vi "svx_Colormap Property Dialog.vi"(5 "Color Map in":refnum<vi>, 6 "Action In":T4, 7 "Refnum":refnum<vi>, 8 "Cursor Lines only?":bool, 9 "Found Speed":bool, 10 "Data In":T2 {"Y scale"."multiplier" format="%.2f"; "Y scale"."offset" format="%.2f"; "X scale"."multiplier" format="%.2f"; "X scale"."offset" format="%.2f"; "spectral map" format="%.2f"}, 11 "State in":T1={"RefQueue"=refnum, "Properties/Undo"=refnum, "Bound"={"Width"=0, "Height"=0}, "Plot Area:Colors"={"FG Color"=11776947, "BG Color"=0}, "scale legend visible?"=FALSE, "graph palette visible?"=FALSE, "cursor palette visible?"=FALSE, "Ignore Array"=TRUE, "Smooth Update"=FALSE, "Z Scale"={"Z Scale.Scale Fit"=2, "Z Scale.Name Label.Text"="Amplitude", "Z Scale.Interpolate Color"=TRUE, "Visible"=TRUE, "Label Visible"=TRUE, "format string"="%#.2g", "Z Scale.Range"={"Minimum"=0.0, "Maximum"=500.0}}, "X Scale"={"X Scale.Scale Fit"=2, "X Scale.Offset and Multiplier"={"Offset"=0.0, "Multiplier"=1.0}, "X Scale.Name Label.Text"="Time", "X Scale.Range"={"Minimum"=0.0, "Maximum"=10.0}, "Visible"=TRUE, "Label Visible"=TRUE, "format string"="%#.2g"}, "Y Scale"={"Y Scale.Scale Fit"=2, "Y Scale.Offset and Multiplier"={"Offset"=0.0, "Multiplier"=1.0}, "Y Scale.Name Label.Text"="Frequency", "Y Scale.Range"={"Minimum"=0.0, "Maximum"=500.0}, "Visible"=TRUE, "Label Visible"=TRUE, "format string"="%#.2g"}, "Annotation List"=[], "Cursor List"=[], "Display Frequency Lines"=TRUE, "Display Order Lines"=TRUE, "Display Order text"=TRUE, "Display Frequency text"=TRUE, "Order Lineproperty"={"Line"={"Width"=1, "Style"=enum."Dash"}, "color"=0}, "Order Textproperty"={"Test size"=11, "color"=16777222, "background"=16777216}, "Orders"=[], "Frequency"=[], "Frequency Lineproperty"={"Line"={"Width"=1, "Style"=enum."Dash"}, "color"=0}, "Frequency Textproperty"={"Test size"=11, "color"=16777222, "background"=16777216}, "Display Order from Cursor"=FALSE, "Display Freq from Cursor"=FALSE, "Active Cursor"=0, "Selected Cursors"=[], "Cursor Move"=refnum, "Scale Range Change"=refnum}) -> (3 "State out":T1={"RefQueue"=refnum, "Properties/Undo"=refnum, "Bound"={"Width"=0, "Height"=0}, "Plot Area:Colors"={"FG Color"=11776947, "BG Color"=0}, "scale legend visible?"=FALSE, "graph palette visible?"=FALSE, "cursor palette visible?"=FALSE, "Ignore Array"=TRUE, "Smooth Update"=FALSE, "Z Scale"={"Z Scale.Scale Fit"=2, "Z Scale.Name Label.Text"="Amplitude", "Z Scale.Interpolate Color"=TRUE, "Visible"=TRUE, "Label Visible"=TRUE, "format string"="%#.2g", "Z Scale.Range"={"Minimum"=0.0, "Maximum"=500.0}}, "X Scale"={"X Scale.Scale Fit"=2, "X Scale.Offset and Multiplier"={"Offset"=0.0, "Multiplier"=1.0}, "X Scale.Name Label.Text"="Time", "X Scale.Range"={"Minimum"=0.0, "Maximum"=10.0}, "Visible"=TRUE, "Label Visible"=TRUE, "format string"="%#.2g"}, "Y Scale"={"Y Scale.Scale Fit"=2, "Y Scale.Offset and Multiplier"={"Offset"=0.0, "Multiplier"=1.0}, "Y Scale.Name Label.Text"="Frequency", "Y Scale.Range"={"Minimum"=0.0, "Maximum"=500.0}, "Visible"=TRUE, "Label Visible"=TRUE, "format string"="%#.2g"}, "Annotation List"=[], "Cursor List"=[], "Display Frequency Lines"=TRUE, "Display Order Lines"=TRUE, "Display Order text"=TRUE, "Display Frequency text"=TRUE, "Order Lineproperty"={"Line"={"Width"=1, "Style"=enum."Dash"}, "color"=0}, "Order Textproperty"={"Test size"=11, "color"=16777222, "background"=16777216}, "Orders"=[], "Frequency"=[], "Frequency Lineproperty"={"Line"={"Width"=1, "Style"=enum."Dash"}, "color"=0}, "Frequency Textproperty"={"Test size"=11, "color"=16777222, "background"=16777216}, "Display Order from Cursor"=FALSE, "Display Freq from Cursor"=FALSE, "Active Cursor"=0, "Selected Cursors"=[], "Cursor Move"=refnum, "Scale Range Change"=refnum}, 4 "Action":T4)   [LabVIEW 2017, in "SVX Colormap.xctl"]
uses:
  <vilib>/addons/_XControls/Colormap/SVX Colormap.xctl
  <vilib>/_xctls/Action.ctl
  <vilib>/addons/_XControls/Colormap/subVIs/svx_Colormap Data.ctl
  <vilib>/addons/_XControls/Colormap/subVIs/svx_Colormap State.ctl
  <vilib>/addons/_XControls/Colormap/TypeDef/svx_Colormap_InnerState.ctl
  <vilib>/addons/_XControls/Colormap/TypeDef/svx_Colormap_Event.ctl
  <vilib>/_xctls/XControlSupport.lvlib
panel:
  in  "Autoscale flag":bool
  in  "Menu":T3(array[cluster])=[{"menu tag"="", "item names"="Delete Element", "item tags"="USER_SC_DELETE_ELEMENT"}, {"menu tag"="", "item names"="Delete All", "item tags"="USER_SC_DELETE_ALL"}]
  in  "Main Tab":T5(tab)
  in  "Enable State":T6(radio)
  in  "Caption":string="Colormap"
  in  "Label Text":string="Colormap"
  in  "Caption":bool
  in  "Label":bool=TRUE
  in  "Apply to":u16(ring) items=["X-Axis", "Y-Axis", "Z-Axis"]
  in  "Hide trailing zeros":bool
  in  "Digits":u8=1
  in  "Precision Type":u16(ring) items=["Digits of precision", "Significant digits"]
  in  "Type":i32(listbox)
  in  "Show scale":bool
  in  "Show scale label":bool
  in  "Axes":u16(ring) items=["X-Axis", "Y-Axis", "Z-Axis"]
  in  "Interpolate color":bool
  in  "Maximum":dbl
  in  "Minimum":dbl
  in  "Autoscale":bool
  in  "Name":string="Time"
  in  "Frequencies":dbl[](array[numeric])
  in  "Orders":dbl[](array[numeric])
  in  "Line Type":u16(ring) items=["Order Lines", "Frequency Lines"]
  in  "DisplayLines":bool
  in  "Displaytext":bool
  in  "Style":T7(ring)=enum."Dash"
  in  "Line width":u16=1 min=1
  in  "Line color":u32(colorbox)
  in  "Size":i16=10 min=1
  in  "Text color":u32(colorbox)=16777222
  in  "BG color":u32(colorbox)=16777216
  in  "Tip strip":string
  in  "Description":string
  in  "Help":bool
  in  "Cancel":bool
  in  "OK":bool
  # "Label"
  # "Caption"
  # "Enabled State"
  # "Line Settings"
  # "Text Settings"
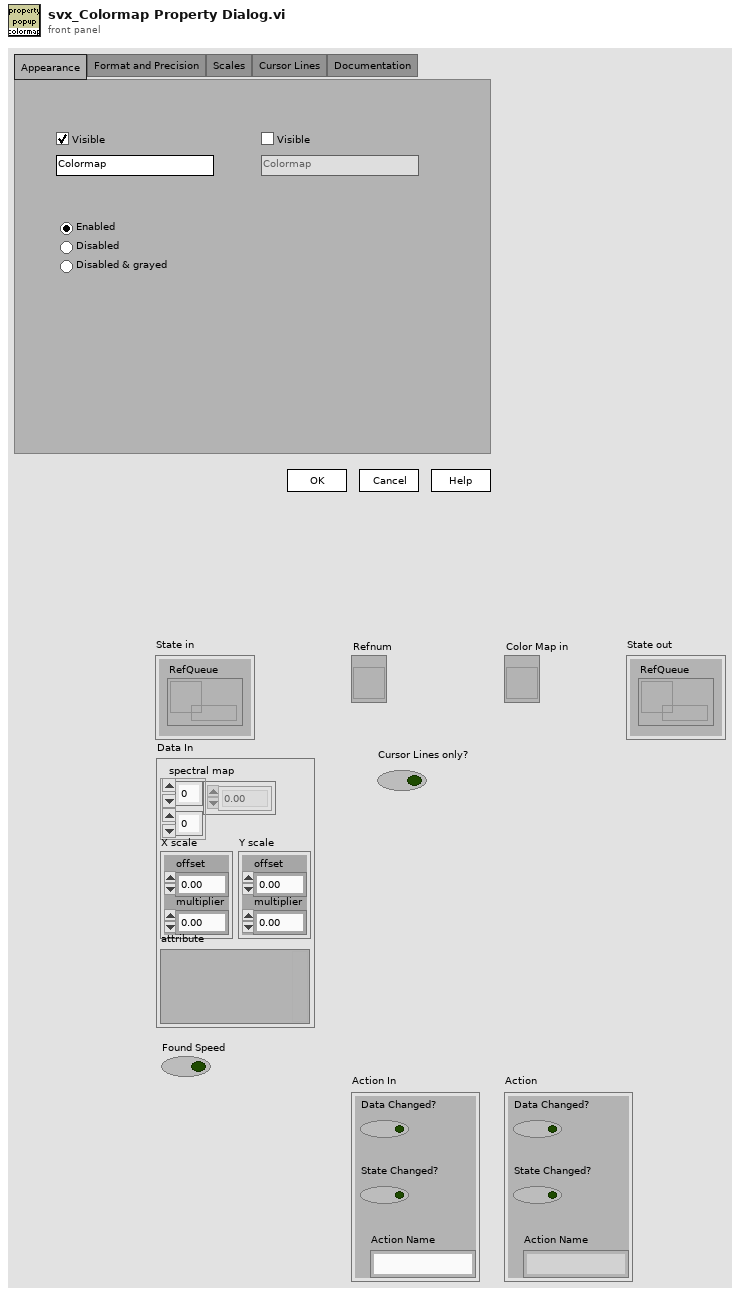
[diagram p1: front panel]
types:
  T1 = typedef "SVX Colormap.xctl/svx_Colormap State.ctl" = cluster{"RefQueue":refnum<queue>, "Properties/Undo":refnum<queue>, "Bound":cluster{"Width":u32, "Height":u32}, "Plot Area:Colors":cluster{"FG Color":u32, "BG Color":u32}, "scale legend visible?":bool, "graph palette visible?":bool, "cursor palette visible?":bool, "Ignore Array":bool, "Smooth Update":bool, "Z Scale":cluster{"Z Scale.Scale Fit":u8, "Z Scale.Name Label.Text":string, "Z Scale.Interpolate Color":bool, "Visible":bool, "Label Visible":bool, "format string":string, "Z Scale.Range":cluster{"Minimum":dbl, "Maximum":dbl}}, "X Scale":cluster{"X Scale.Scale Fit":u8, "X Scale.Offset and Multiplier":cluster{"Offset":dbl, "Multiplier":dbl}, "X Scale.Name Label.Text":string, "X Scale.Range":cluster{"Minimum":dbl, "Maximum":dbl}, "Visible":bool, "Label Visible":bool, "format string":string}, "Y Scale":cluster{"Y Scale.Scale Fit":u8, "Y Scale.Offset and Multiplier":cluster{"Offset":dbl, "Multiplier":dbl}, "Y Scale.Name Label.Text":string, "Y Scale.Range":cluster{"Minimum":dbl, "Maximum":dbl}, "Visible":bool, "Label Visible":bool, "format string":string}, "Annotation List":cluster{"Name":string, "Color":u32, "Style":u8, "Point Style":u8, "Name Visible":bool, "Allow Drag":bool, "Annotation Mode":u32, "Plot":i32, "Index":i32, "Position":cluster{"X":dbl, "Y":dbl}, "X Scale":u32, "Y Scale":u32, "Show Arrow":bool, "Lock Name":bool, "Plot Area":i32, "Label Offset":cluster{"X":dbl, "Y":dbl}}[], "Cursor List":cluster{"Name":string, "Color":u32, "Style":u8, "Point Style":u8, "Name Visible":bool, "Allow Drag":bool, "Cursor Mode":u32, "Plot":i32, "Index":i32, "Position":cluster{"X":dbl, "Y":dbl}, "X Scale":u32, "Y Scale":u32, "Watch Plots":i32[], "Watch All Plots":bool, "Plot Area":i32, "Label Offset":cluster{"X":dbl, "Y":dbl}}[], "Display Frequency Lines":bool, "Display Order Lines":bool, "Display Order text":bool, "Display Frequency text":bool, "Order Lineproperty":cluster{"Line":cluster{"Width":u16, "Style":enum32{"Solid", "Dash", "Dot", "DashDot", "DashDotDot"}}, "color":u32}, "Order Textproperty":cluster{"Test size":i16, "color":u32, "background":u32}, "Orders":dbl[], "Frequency":dbl[], "Frequency Lineproperty":cluster{"Line":cluster{"Width":u16, "Style":enum32{"Solid", "Dash", "Dot", "DashDot", "DashDotDot"}}, "color":u32}, "Frequency Textproperty":cluster{"Test size":i16, "color":u32, "background":u32}, "Display Order from Cursor":bool, "Display Freq from Cursor":bool, "Active Cursor":u32, "Selected Cursors":u32[], "Cursor Move":refnum<user-event>, "Scale Range Change":refnum<user-event>}
  T2 = typedef "SVX Colormap.xctl/svx_Colormap Data.ctl" = cluster{"spectral map":dbl[][], "X scale":cluster{"offset":dbl, "multiplier":dbl}, "Y scale":cluster{"offset":dbl, "multiplier":dbl}, "attribute":variant}
  T3 = cluster{"menu tag":string, "item names":string, "item tags":string}[]
  T4 = typedef "XControlSupport.lvlib/Action.ctl" = cluster{"Data Changed?":bool, "State Changed?":bool, "Action Name":string}
  T5 = enum32{"Appearance", "Format and Precision", "Scales", "Cursor Lines", "Documentation"}
  T6 = enum32{"Enabled", "Disabled", "Disabled & grayed"}
  T7 = enum32{"Solid", "Dash", "Dot", "DashDot", "DashDotDot"}
  T8 = cluster{"Label.Text":string, "Caption.Text":string, "Label.Visible":bool, "Caption.Visible":bool, "Disabled":u8, "Desc":string, "TipStrip":string}
  T9 = cluster{"Test size":i16, "color":u32, "background":u32}
  T10 = cluster{"Line":cluster{"Width":u16, "Style":enum32{"Solid", "Dash", "Dot", "DashDot", "DashDotDot"}}, "color":u32}
  T11 = typedef "SVX Colormap.xctl/svx_Colormap_Event.ctl" = enum16{"None", "[Axis] X Range", "[Axis] Y Range", "[Axis] Z Range", "[Axis] Range", "[Axis] X FString", "[Axis] Y FString", "[Axis] Z FString", "[Axis] X Name", "[Axis] X ScaleVis", "[Axis] X NameVis", "[Axis] Y Name", "[Axis] Y ScaleVis", "[Axis] Y NameVis", "[Axis] Z Name", "[Axis] Z ScaleVis", "[Axis] Z NameVis", "[Image] Line", "[Axis] Z Interp", "[Data] Update", "[Layout] Resize", "[ColorTable] Ignore Array", "[Legend] ScaleVis", "[Legend] GPVis", "[Legend] CPVis", "[Smooth] Update", "[Cursor] Update", "[Plot Area] Colors", "[Size] Minimum", "[Annotation] Update", "[Properties Dialog]", "[Axis] Autoscale X", "[Axis] Autoscale Y", "[Axis] Autoscale Z"}
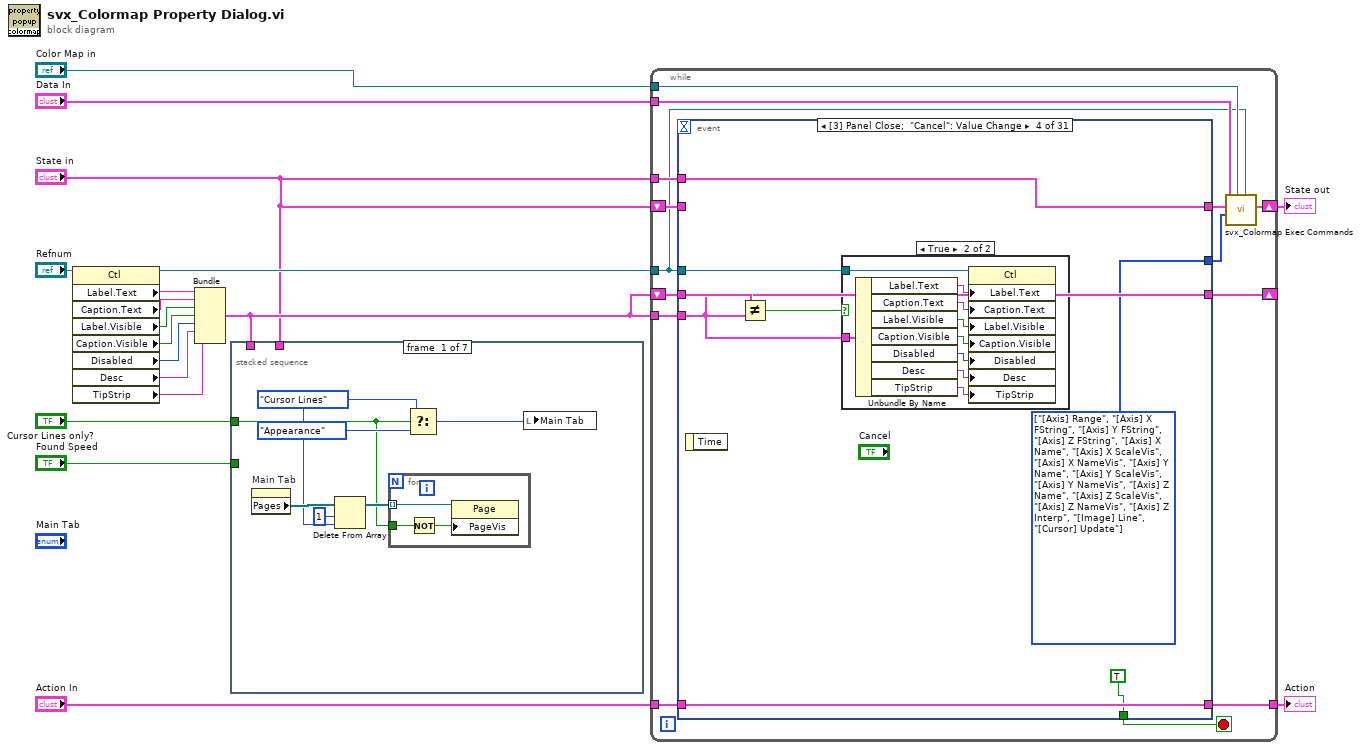
[diagram p0: block diagram]
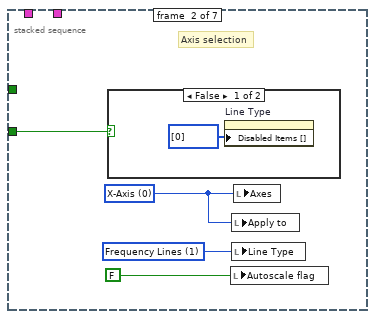
[diagram p2: hidden frame]
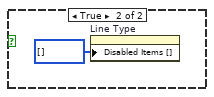
[diagram p3: hidden frame]
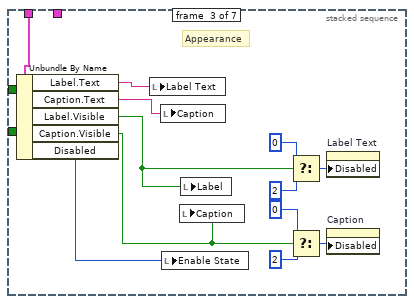
[diagram p4: hidden frame]
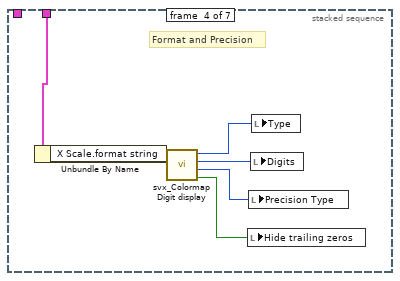
[diagram p5: hidden frame]
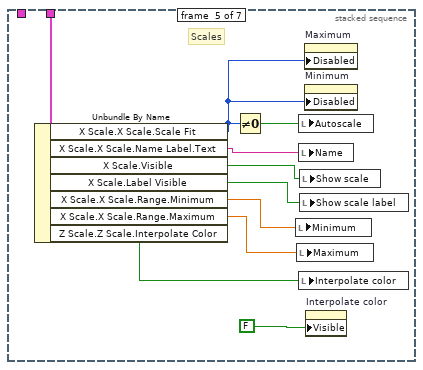
[diagram p6: hidden frame]
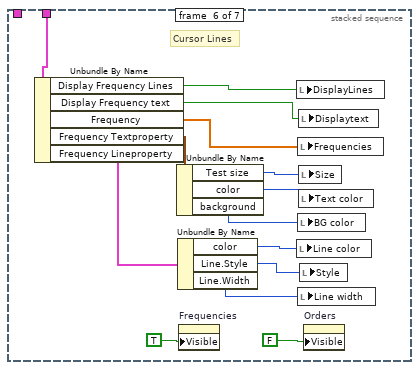
[diagram p7: hidden frame]
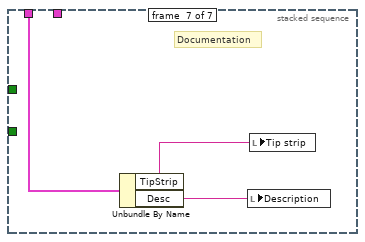
[diagram p8: hidden frame]
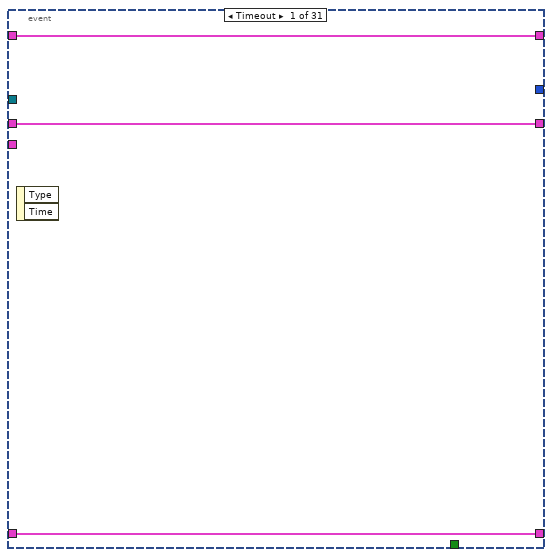
[diagram p9: hidden frame]
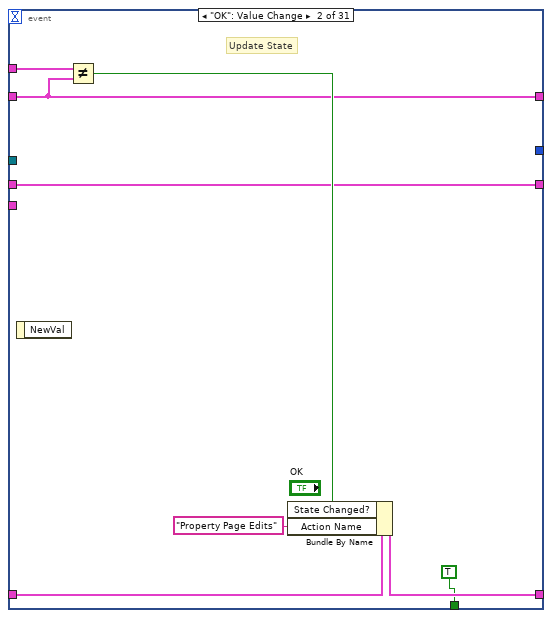
[diagram p10: hidden frame]
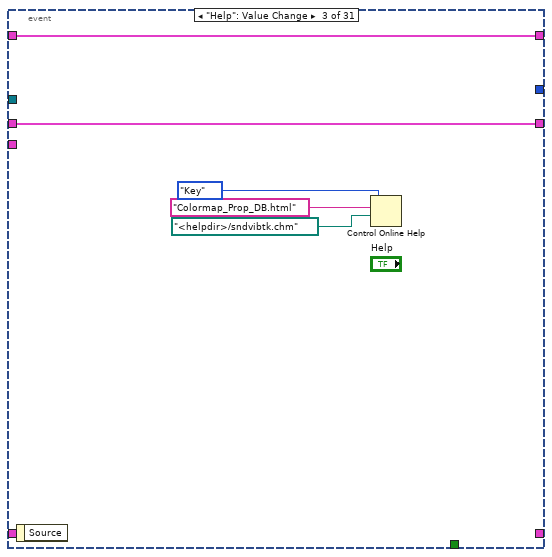
[diagram p11: hidden frame]
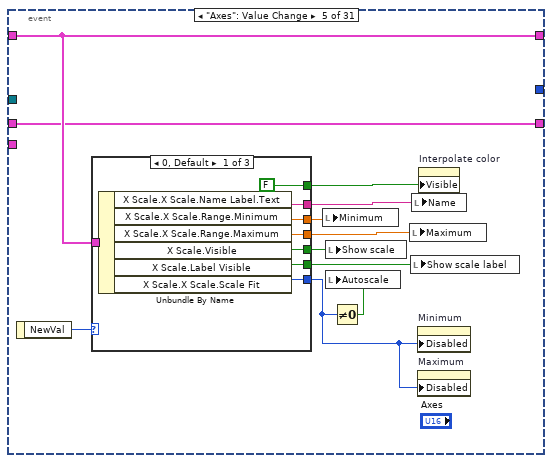
[diagram p13: hidden frame]
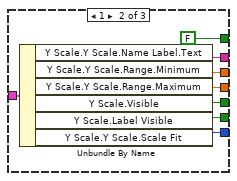
[diagram p14: hidden frame]
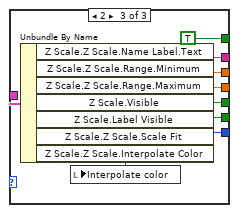
[diagram p15: hidden frame]
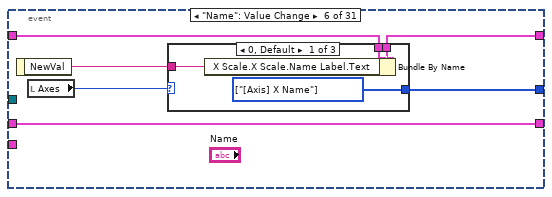
[diagram p16: hidden frame]
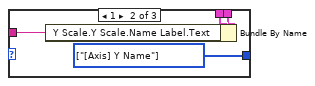
[diagram p17: hidden frame]
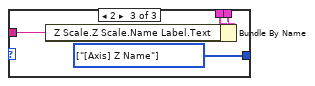
[diagram p18: hidden frame]
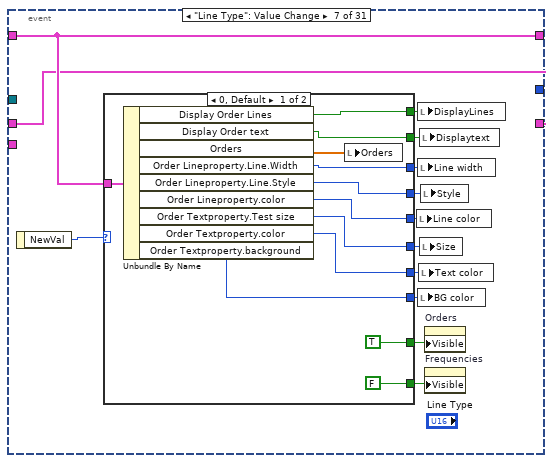
[diagram p19: hidden frame]
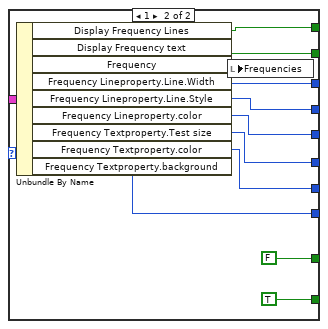
[diagram p20: hidden frame]
diagram:
  n1 = property class="Ctl"(reference="Refnum") -> (reference out=w14:refnum<vi>, "Label.Text"=w13:string, "Caption.Text"=w12:string, "Label.Visible"=w11:bool, "Caption.Visible"=w10:bool, "Disabled"=w9:u8, "Desc"=w8:string, "TipStrip"=w7:string)  [unwired: 1 in, 1 out]
  n2 = Bundle("Label.Text"=w13, "Caption.Text"=w12, "Label.Visible"=w11, "Caption.Visible"=w10, "Disabled"=w9, "Desc"=w8, "TipStrip"=w7) -> (w5:T8)  [unwired: 1 in]
  n3 = stacked-sequence {
    tunnel: "State in" -> [_ _ _ w51 w62 w74 _]
    tunnel: w5 -> [_ _ w40 _ _ _ w77]
    tunnel: "Found Speed" -> [_ w30 _ _ _ _ _]
    tunnel: "Cursor Lines only?" -> [w19 _ _ _ _ _ _]
    frame #0 {
      w22 = T5."Cursor Lines" ("Main Tab")
      n4 = property on="Main Tab" class="TabCtl (strict)"() -> ("Pages"=w23:refnum<vi>[])  [unwired: 2 in, 2 out]
      n5 = Delete From Array(array=w23, length=1, index=w22) -> (array with subset deleted=w20:refnum<vi>[])  [unwired: 1 out]
      n6 = for {
        tunnel: w20 -> [w28] mode=indexing
        tunnel: w19 -> [w26]
        n7 = Not(x=w26) -> (.not. x?=w27:bool)
        n8 = property class="Page"(reference=w28, "PageVis"=w27) -> ()  [unwired: 1 in, 2 out]
      }
      n9 = Select(t=w22, s=w19, f=T5."Appearance") -> (s? t:f=w25:T5)
      n10 = local write "Main Tab"(w25) -> ()
    }
    frame #1 {
      w31 = u16 1 items=["Order Lines", "Frequency Lines"] ("line selection")
      w32 = u16 0 items=["X-Axis", "Y-Axis", "Z-Axis"] ("axis selection")
      # "Axis selection"
      n11 = case shown="False" w30 {
        frame False {
          n12 = property on="Line Type" class="Ring (strict)"("Disabled Items []"=i32[] [0]) -> ()  [unwired: 2 in, 2 out]
        }
        frame True {
          n13 = property on="Line Type" class="Ring (strict)"("Disabled Items []"=i32[] []) -> ()  [unwired: 2 in, 2 out]
        }
      }
      n14 = local write "Autoscale flag"(FALSE ("Autoscale flag")) -> ()
      n15 = local write "Apply to"(w32) -> ()
      n16 = local write "Line Type"(w31) -> ()
      n17 = local write "Axes"(w32) -> ()
    }
    frame #2 {
      # "Appearance"
      n18 = Unbundle By Name(w40) -> ("Label.Text"=w39:string, "Caption.Text"=w38:string, "Label.Visible"=w37:bool, "Caption.Visible"=w36:bool, "Disabled"=w35:u8)
      n19 = local write "Label Text"(w39) -> ()
      n20 = local write "Caption"(w38) -> ()
      n21 = local write "Enable State"(w35) -> ()
      n22 = local write "Caption"(w36) -> ()
      n23 = local write "Label"(w37) -> ()
      n24 = Select(t=u8 0, s=w37, f=u8 2) -> (s? t:f=w42:u8)
      n25 = Select(t=u8 0 ("Disabled"), s=w36, f=u8 2) -> (s? t:f=w43:u8)
      n26 = property on="Label Text" class="Str"("Disabled"=w42) -> ()  [unwired: 2 in, 2 out]
      n27 = property on="Caption" class="Str"("Disabled"=w43) -> ()  [unwired: 2 in, 2 out]
    }
    frame #3 {
      # "Format and Precision"
      n28 = Unbundle By Name(w51) -> ("X Scale.format string"=w50:string)
      n29 = call <vilib>:"svx_Colormap Digit display.vi"("Format string"=w50) -> ("trailing zeros"=w47:bool, "Precision Type"=w48:u16, "Digits"=w49:u8, "Type"=w52:i32)  [unwired: 7 in]
      n30 = local write "Hide trailing zeros"(w47) -> ()
      n31 = local write "Precision Type"(w48) -> ()
      n32 = local write "Digits"(w49) -> ()
      n33 = local write "Type"(w52) -> ()
    }
    frame #4 {
      # "Scales"
      n34 = Unbundle By Name(w62) -> ("X Scale.X Scale.Scale Fit"=w53:u8, "X Scale.X Scale.Name Label.Text"=w61:string, "X Scale.Visible"=w60:bool, "X Scale.Label Visible"=w59:bool, "X Scale.X Scale.Range.Minimum"=w58:dbl, "X Scale.X Scale.Range.Maximum"=w57:dbl, "Z Scale.Z Scale.Interpolate Color"=w55:bool)
      n35 = Not Equal To 0?(x=w53) -> (x != 0?=w54:bool)
      n36 = local write "Minimum"(w58) -> ()
      n37 = local write "Maximum"(w57) -> ()
      n38 = local write "Autoscale"(w54) -> ()
      n39 = local write "Name"(w61) -> ()
      n40 = local write "Interpolate color"(w55) -> ()
      n41 = local write "Show scale"(w60) -> ()
      n42 = local write "Show scale label"(w59) -> ()
      n43 = property on="Maximum" class="DigNum (strict)"("Disabled"=w53) -> ()  [unwired: 2 in, 2 out]
      n44 = property on="Minimum" class="DigNum (strict)"("Disabled"=w53) -> ()  [unwired: 2 in, 2 out]
      n45 = property on="Interpolate color" class="Bool (strict)"("Visible"=FALSE) -> ()  [unwired: 2 in, 2 out]
    }
    frame #5 {
      # "Cursor Lines"
      n46 = Unbundle By Name(w74) -> ("Display Frequency Lines"=w73:bool, "Display Frequency text"=w72:bool, "Frequency"=w64:dbl[], "Frequency Textproperty"=w71:T9, "Frequency Lineproperty"=w70:T10)
      n47 = Unbundle By Name(w71) -> ("Test size"=w75:i16, "color"=w69:u32, "background"=w68:u32)
      n48 = Unbundle By Name(w70) -> ("color"=w76:u32, "Line.Style"=w66:T7, "Line.Width"=w67:u16)
      n49 = property on="Frequencies" class="Arr (strict)"("Visible"=TRUE) -> ()  [unwired: 2 in, 2 out]
      n50 = local write "DisplayLines"(w73) -> ()
      n51 = local write "Line color"(w76) -> ()
      n52 = local write "Frequencies"(w64) -> ()
      n53 = local write "BG color"(w68) -> ()
      n54 = local write "Line width"(w67) -> ()
      n55 = local write "Displaytext"(w72) -> ()
      n56 = local write "Size"(w75) -> ()
      n57 = local write "Text color"(w69) -> ()
      n58 = local write "Style"(w66) -> ()
      n59 = property on="Orders" class="Arr (strict)"("Visible"=FALSE) -> ()  [unwired: 2 in, 2 out]
    }
    frame #6 {
      # "Documentation"
      n60 = Unbundle By Name(w77) -> ("TipStrip"=w78:string, "Desc"=w79:string)
      n61 = local write "Description"(w79) -> ()
      n62 = local write "Tip strip"(w78) -> ()
    }
  }
  n63 = while {
    shift-right: [w85] -> w2
    shift-left: "State in" -> [w90]
    tunnel: w14 -> [w80]
    tunnel: "Color Map in" -> [w84]
    tunnel: "State in" -> [w91]
    shift-right: [w87] -> _
    shift-left: w5 -> [w81]
    tunnel: w5 -> [w88]
    tunnel: "Data In" -> [w83]
    tunnel: "Action In" -> [w92]
    tunnel: [w89] -> w16
    stop <- w93 stop-if-true
    n64 = event shown="[3] Panel Close;  \"Cancel\": Value Change" {
      selector: _ -> [_ _ _ _ _ _ _ _ _ _ _ _ _ _ _ _ _ _ _ _ _ _ _ _ _ _ _ _ _ _ _]
      dyn-events: _ -> [_ _ _ _ _ _ _ _ _ _ _ _ _ _ _ _ _ _ _ _ _ _ _ _ _ _ _ _ _ _ _]
      timeout: _ -> [_ _ _ _ _ _ _ _ _ _ _ _ _ _ _ _ _ _ _ _ _ _ _ _ _ _ _ _ _ _ _]
      tunnel: w90 -> [w96 w98 w105 _ w130 w168 w184 w223 w244 w260 w284 w294 w303 w322 w324 w336 w354 w358 w370 w381 w402 w423 w443 w447 w455 w460 w468 w473 w479 w484 w496]
      tunnel: [_ TRUE _ TRUE _ _ _ _ _ _ _ _ _ _ _ _ _ _ _ _ _ _ _ _ _ _ _ _ _ _ _] -> w93
      tunnel: w80 -> [_ _ _ w113 _ _ _ _ _ _ _ _ _ _ _ _ _ _ _ _ _ _ _ w448 w456 w461 w469 w474 w480 w485 _]
      tunnel: w92 -> [w95 w104 _ w117 _ _ _ _ _ _ _ _ _ _ _ _ _ _ _ _ _ _ _ _ _ _ _ _ _ _ _]
      tunnel: [w95 w103 _ w117 _ _ _ _ _ _ _ _ _ _ _ _ _ _ _ _ _ _ _ _ _ _ _ _ _ _ _] -> w89
      tunnel: [w96 w98 w105 w115 w130 w167 w184 w222 w242 w259 w284 w294 w302 w320 w324 w334 w352 w357 w369 w380 w401 w422 w442 w447 w455 w460 w468 w473 w479 w484 w495] -> w86
      tunnel: w91 -> [_ w100 _ w115 _ _ _ _ _ _ _ _ _ _ _ _ _ _ _ _ _ _ _ _ _ _ _ _ _ _ _]
      tunnel: w88 -> [_ _ _ w111 _ _ _ _ _ _ _ _ _ _ _ _ _ _ _ _ _ _ _ _ _ _ _ _ _ _ _]
      tunnel: [w94 w97 w106 w111 w129 w164 w181 w224 w239 w256 w277 w291 w306 w319 w323 w337 w351 w360 w372 w382 w398 w420 w440 w445 w453 w458 w466 w470 w477 w482 w492] -> w87
      tunnel: [_ _ _ w110 _ w163 _ w219 _ w257 _ _ w305 w318 _ w338 w350 w359 w371 w379 w399 w421 w439 _ _ _ _ _ _ _ w494] -> w82
      tunnel: w81 -> [w94 w97 w106 w114 w129 w164 w181 w224 w239 w256 w277 w291 w306 w319 w323 w337 w351 w360 w372 w382 w398 w420 w440 w446 w454 w459 w467 w472 w478 w483 w492]
      event Timeout {
        n65 = event-data() -> ()  [unwired: 1 in, 2 out]
      }
      event "OK": Value Change {
        # "Update State"
        n66 = event-data() -> ()  [unwired: 1 in, 1 out]
        n67 = Not Equal?(x=w100, y=w98) -> (x != y?=w99:bool)
        n68 = Bundle By Name(cluster=w104, "State Changed?"=w99, "Action Name"="Property Page Edits") -> (w103:T4)
      }
      event "Help": Value Change {
        n69 = event-data() -> ()  [unwired: 1 in, 1 out]
        n70 = Control Online Help(2:path "<helpdir>/sndvibtk.chm" ("Path to the help file"), 3:"Colormap_Prop_DB.html" ("String to search for"), 4:enum16{"Contents", "Key", "Close"}."Key" ("Operation")) -> ()  [unwired: 1 in, 1 out]
      }
      event Panel Close; "Cancel": Value Change {
        w110 = T11[] [enum."[Axis] Range", enum."[Axis] X FString", enum."[Axis] Y FString", enum."[Axis] Z FString", enum."[Axis] X Name", enum."[Axis] X ScaleVis", enum."[Axis] X NameVis", enum."[Axis] Y Name", enum."[Axis] Y ScaleVis", enum."[Axis] Y NameVis", enum."[Axis] Z Name", enum."[Axis] Z ScaleVis", enum."[Axis] Z NameVis", enum."[Axis] Z Interp", enum."[Image] Line", enum."[Cursor] Update"] items=["None", "[Axis] X Range", "[Axis] Y Range", "[Axis] Z Range", "[Axis] Range", "[Axis] X FString", "[Axis] Y FString", "[Axis] Z FString", "[Axis] X Name", "[Axis] X ScaleVis", "[Axis] X NameVis", "[Axis] Y Name", "[Axis] Y ScaleVis", "[Axis] Y NameVis", "[Axis] Z Name", "[Axis] Z ScaleVis", "[Axis] Z NameVis", "[Image] Line", "[Axis] Z Interp", "[Data] Update", "[Layout] Resize", "[ColorTable] Ignore Array", "[Legend] ScaleVis", "[Legend] GPVis", "[Legend] CPVis", "[Smooth] Update", "[Cursor] Update", "[Plot Area] Colors", "[Size] Minimum", "[Annotation] Update", "[Properties Dialog]", "[Axis] Autoscale X", "[Axis] Autoscale Y", "[Axis] Autoscale Z"] ("remaining elements")
        n71 = event-data() -> ()  [unwired: 1 in, 1 out]
        n72 = Not Equal?(x=w114, y=w111) -> (x != y?=w112:bool)
        n73 = case shown="True" w112 {
          tunnel: w113 -> [_ w126]
          tunnel: w111 -> [_ w125]
          frame False {
          }
          frame True {
            n74 = Unbundle By Name(w125) -> ("Label.Text"=w124:string, "Caption.Text"=w123:string, "Label.Visible"=w122:bool, "Caption.Visible"=w121:bool, "Disabled"=w120:u8, "Desc"=w119:string, "TipStrip"=w118:string)
            n75 = property class="Ctl"(reference=w126, "Label.Text"=w124, "Caption.Text"=w123, "Label.Visible"=w122, "Caption.Visible"=w121, "Disabled"=w120, "Desc"=w119, "TipStrip"=w118) -> ()  [unwired: 1 in, 2 out]
          }
        }
      }
      event "Axes": Value Change {
        n76 = event-data() -> ("NewVal"=w137:u16)  [unwired: 1 in]
        n77 = case shown="0, Default" w137 {
          tunnel: [w145 w153 w162] -> w135
          tunnel: [w138 w146 w155] -> w128
          tunnel: [w144 w152 w159] -> w134
          tunnel: [w143 w151 w158] -> w133
          tunnel: [w142 w150 w160] -> w132
          tunnel: [w141 w149 w161] -> w131
          tunnel: [FALSE ("Visible") FALSE ("Visible") TRUE ("Visible")] -> w136
          tunnel: w130 -> [w139 w147 w156]
          frame 0, Default {
            n78 = Unbundle By Name(w139) -> ("X Scale.X Scale.Name Label.Text"=w145:string, "X Scale.X Scale.Range.Minimum"=w144:dbl, "X Scale.X Scale.Range.Maximum"=w143:dbl, "X Scale.Visible"=w142:bool, "X Scale.Label Visible"=w141:bool, "X Scale.X Scale.Scale Fit"=w138:u8)
          }
          frame 1 {
            n79 = Unbundle By Name(w147) -> ("Y Scale.Y Scale.Name Label.Text"=w153:string, "Y Scale.Y Scale.Range.Minimum"=w152:dbl, "Y Scale.Y Scale.Range.Maximum"=w151:dbl, "Y Scale.Visible"=w150:bool, "Y Scale.Label Visible"=w149:bool, "Y Scale.Y Scale.Scale Fit"=w146:u8)
          }
          frame 2 {
            n80 = Unbundle By Name(w156) -> ("Z Scale.Z Scale.Name Label.Text"=w162:string, "Z Scale.Z Scale.Range.Minimum"=w159:dbl, "Z Scale.Z Scale.Range.Maximum"=w158:dbl, "Z Scale.Visible"=w160:bool, "Z Scale.Label Visible"=w161:bool, "Z Scale.Z Scale.Scale Fit"=w155:u8, "Z Scale.Z Scale.Interpolate Color"=w154:bool)
            n81 = local write "Interpolate color"(w154) -> ()
          }
        }
        n82 = local write "Minimum"(w134) -> ()
        n83 = local write "Show scale"(w132) -> ()
        n84 = Not Equal To 0?(x=w128) -> (x != 0?=w127:bool)
        n85 = local write "Autoscale"(w127) -> ()
        n86 = local write "Maximum"(w133) -> ()
        n87 = local write "Show scale label"(w131) -> ()
        n88 = local write "Name"(w135) -> ()
        n89 = property on="Minimum" class="DigNum (strict)"("Disabled"=w128) -> ()  [unwired: 2 in, 2 out]
        n90 = property on="Maximum" class="DigNum (strict)"("Disabled"=w128) -> ()  [unwired: 2 in, 2 out]
        n91 = property on="Interpolate color" class="Bool (strict)"("Visible"=w136) -> ()  [unwired: 2 in, 2 out]
      }
      event "Name": Value Change {
        n92 = event-data() -> ("NewVal"=w166:string)  [unwired: 1 in]
        n93 = local read "Axes"() -> (w165:u16)
        n94 = case shown="0, Default" w165 {
          tunnel: w168 -> [w172 w176 w180]
          tunnel: [w171 w175 w179] -> w167
          tunnel: w166 -> [w170 w174 w178]
          tunnel: [w169 w173 w177] -> w163
          frame 0, Default {
            w169 = T11[] [enum."[Axis] X Name"] items=["None", "[Axis] X Range", "[Axis] Y Range", "[Axis] Z Range", "[Axis] Range", "[Axis] X FString", "[Axis] Y FString", "[Axis] Z FString", "[Axis] X Name", "[Axis] X ScaleVis", "[Axis] X NameVis", "[Axis] Y Name", "[Axis] Y ScaleVis", "[Axis] Y NameVis", "[Axis] Z Name", "[Axis] Z ScaleVis", "[Axis] Z NameVis", "[Image] Line", "[Axis] Z Interp", "[Data] Update", "[Layout] Resize", "[ColorTable] Ignore Array", "[Legend] ScaleVis", "[Legend] GPVis", "[Legend] CPVis", "[Smooth] Update", "[Cursor] Update", "[Plot Area] Colors", "[Size] Minimum", "[Annotation] Update", "[Properties Dialog]", "[Axis] Autoscale X", "[Axis] Autoscale Y", "[Axis] Autoscale Z"] ("Events")
            n95 = Bundle By Name(cluster=w172, "X Scale.X Scale.Name Label.Text"=w170) -> (w171:T1)
          }
          frame 1 {
            w173 = T11[] [enum."[Axis] Y Name"] items=["None", "[Axis] X Range", "[Axis] Y Range", "[Axis] Z Range", "[Axis] Range", "[Axis] X FString", "[Axis] Y FString", "[Axis] Z FString", "[Axis] X Name", "[Axis] X ScaleVis", "[Axis] X NameVis", "[Axis] Y Name", "[Axis] Y ScaleVis", "[Axis] Y NameVis", "[Axis] Z Name", "[Axis] Z ScaleVis", "[Axis] Z NameVis", "[Image] Line", "[Axis] Z Interp", "[Data] Update", "[Layout] Resize", "[ColorTable] Ignore Array", "[Legend] ScaleVis", "[Legend] GPVis", "[Legend] CPVis", "[Smooth] Update", "[Cursor] Update", "[Plot Area] Colors", "[Size] Minimum", "[Annotation] Update", "[Properties Dialog]", "[Axis] Autoscale X", "[Axis] Autoscale Y", "[Axis] Autoscale Z"] ("Events")
            n96 = Bundle By Name(cluster=w176, "Y Scale.Y Scale.Name Label.Text"=w174) -> (w175:T1)
          }
          frame 2 {
            w177 = T11[] [enum."[Axis] Z Name"] items=["None", "[Axis] X Range", "[Axis] Y Range", "[Axis] Z Range", "[Axis] Range", "[Axis] X FString", "[Axis] Y FString", "[Axis] Z FString", "[Axis] X Name", "[Axis] X ScaleVis", "[Axis] X NameVis", "[Axis] Y Name", "[Axis] Y ScaleVis", "[Axis] Y NameVis", "[Axis] Z Name", "[Axis] Z ScaleVis", "[Axis] Z NameVis", "[Image] Line", "[Axis] Z Interp", "[Data] Update", "[Layout] Resize", "[ColorTable] Ignore Array", "[Legend] ScaleVis", "[Legend] GPVis", "[Legend] CPVis", "[Smooth] Update", "[Cursor] Update", "[Plot Area] Colors", "[Size] Minimum", "[Annotation] Update", "[Properties Dialog]", "[Axis] Autoscale X", "[Axis] Autoscale Y", "[Axis] Autoscale Z"] ("Events")
            n97 = Bundle By Name(cluster=w180, "Z Scale.Z Scale.Name Label.Text"=w178) -> (w179:T1)
          }
        }
      }
      event "Line Type": Value Change {
        n98 = event-data() -> ("NewVal"=w193:u16)  [unwired: 1 in]
        n99 = case shown="0, Default" w193 {
          tunnel: w184 -> [w205 w216]
          tunnel: [w204 w215] -> w192
          tunnel: [w203 w214] -> w191
          tunnel: [w202 w217] -> w190
          tunnel: [w201 w213] -> w189
          tunnel: [w200 w212] -> w188
          tunnel: [w199 w211] -> w187
          tunnel: [w198 w210] -> w186
          tunnel: [w196 w209] -> w185
          tunnel: [FALSE ("Visible") TRUE ("Visible")] -> w183
          tunnel: [TRUE ("Visible") FALSE ("Visible")] -> w182
          frame 0, Default {
            n100 = Unbundle By Name(w205) -> ("Display Order Lines"=w204:bool, "Display Order text"=w203:bool, "Orders"=w197:dbl[], "Order Lineproperty.Line.Width"=w202:u16, "Order Lineproperty.Line.Style"=w201:T7, "Order Lineproperty.color"=w200:u32, "Order Textproperty.Test size"=w199:i16, "Order Textproperty.color"=w198:u32, "Order Textproperty.background"=w196:u32)
            n101 = local write "Orders"(w197) -> ()
          }
          frame 1 {
            n102 = Unbundle By Name(w216) -> ("Display Frequency Lines"=w215:bool, "Display Frequency text"=w214:bool, "Frequency"=w208:dbl[], "Frequency Lineproperty.Line.Width"=w217:u16, "Frequency Lineproperty.Line.Style"=w213:T7, "Frequency Lineproperty.color"=w212:u32, "Frequency Textproperty.Test size"=w211:i16, "Frequency Textproperty.color"=w210:u32, "Frequency Textproperty.background"=w209:u32)
            n103 = local write "Frequencies"(w208) -> ()
          }
        }
        n104 = local write "Line color"(w188) -> ()
        n105 = local write "DisplayLines"(w192) -> ()
        n106 = local write "Line width"(w190) -> ()
        n107 = local write "BG color"(w185) -> ()
        n108 = local write "Text color"(w186) -> ()
        n109 = local write "Displaytext"(w191) -> ()
        n110 = local write "Size"(w187) -> ()
        n111 = local write "Style"(w189) -> ()
        n112 = property on="Orders" class="Arr (strict)"("Visible"=w182) -> ()  [unwired: 2 in, 2 out]
        n113 = property on="Frequencies" class="Arr (strict)"("Visible"=w183) -> ()  [unwired: 2 in, 2 out]
      }
      event "Autoscale": Value Change {
        n114 = event-data() -> ("NewVal"=w218:bool)  [unwired: 1 in]
        n115 = local read "Axes"() -> (w221:u16)
        n116 = Boolean To (0,1)(Boolean=w218) -> (0, 1=w225:i16)
        n117 = Add(x=w225, y=w225) -> (x+y=w220:i16)
        n118 = case shown="True" w218 {
          selector: w218 -> [_ w226]
          frame False {
          }
          frame True {
            n119 = property on="Autoscale flag" class="Bool (strict)"("Val(Sgnl)"=w226) -> ()  [unwired: 2 in, 2 out]
          }
        }
        n120 = case shown="0, Default" w221 {
          tunnel: w223 -> [w230 w234 w238]
          tunnel: [w229 w233 w237] -> w222
          tunnel: w220 -> [w228 w232 w236]
          tunnel: [w227 w231 w235] -> w219
          frame 0, Default {
            w227 = T11[] [enum."[Axis] X Range"] items=["None", "[Axis] X Range", "[Axis] Y Range", "[Axis] Z Range", "[Axis] Range", "[Axis] X FString", "[Axis] Y FString", "[Axis] Z FString", "[Axis] X Name", "[Axis] X ScaleVis", "[Axis] X NameVis", "[Axis] Y Name", "[Axis] Y ScaleVis", "[Axis] Y NameVis", "[Axis] Z Name", "[Axis] Z ScaleVis", "[Axis] Z NameVis", "[Image] Line", "[Axis] Z Interp", "[Data] Update", "[Layout] Resize", "[ColorTable] Ignore Array", "[Legend] ScaleVis", "[Legend] GPVis", "[Legend] CPVis", "[Smooth] Update", "[Cursor] Update", "[Plot Area] Colors", "[Size] Minimum", "[Annotation] Update", "[Properties Dialog]", "[Axis] Autoscale X", "[Axis] Autoscale Y", "[Axis] Autoscale Z"] ("Events")
            n121 = Bundle By Name(cluster=w230, "X Scale.X Scale.Scale Fit"=w228) -> (w229:T1)
          }
          frame 1 {
            w231 = T11[] [enum."[Axis] Y Range"] items=["None", "[Axis] X Range", "[Axis] Y Range", "[Axis] Z Range", "[Axis] Range", "[Axis] X FString", "[Axis] Y FString", "[Axis] Z FString", "[Axis] X Name", "[Axis] X ScaleVis", "[Axis] X NameVis", "[Axis] Y Name", "[Axis] Y ScaleVis", "[Axis] Y NameVis", "[Axis] Z Name", "[Axis] Z ScaleVis", "[Axis] Z NameVis", "[Image] Line", "[Axis] Z Interp", "[Data] Update", "[Layout] Resize", "[ColorTable] Ignore Array", "[Legend] ScaleVis", "[Legend] GPVis", "[Legend] CPVis", "[Smooth] Update", "[Cursor] Update", "[Plot Area] Colors", "[Size] Minimum", "[Annotation] Update", "[Properties Dialog]", "[Axis] Autoscale X", "[Axis] Autoscale Y", "[Axis] Autoscale Z"] ("Events")
            n122 = Bundle By Name(cluster=w234, "Y Scale.Y Scale.Scale Fit"=w232) -> (w233:T1)
          }
          frame 2 {
            w235 = T11[] [enum."[Axis] Z Range"] items=["None", "[Axis] X Range", "[Axis] Y Range", "[Axis] Z Range", "[Axis] Range", "[Axis] X FString", "[Axis] Y FString", "[Axis] Z FString", "[Axis] X Name", "[Axis] X ScaleVis", "[Axis] X NameVis", "[Axis] Y Name", "[Axis] Y ScaleVis", "[Axis] Y NameVis", "[Axis] Z Name", "[Axis] Z ScaleVis", "[Axis] Z NameVis", "[Image] Line", "[Axis] Z Interp", "[Data] Update", "[Layout] Resize", "[ColorTable] Ignore Array", "[Legend] ScaleVis", "[Legend] GPVis", "[Legend] CPVis", "[Smooth] Update", "[Cursor] Update", "[Plot Area] Colors", "[Size] Minimum", "[Annotation] Update", "[Properties Dialog]", "[Axis] Autoscale X", "[Axis] Autoscale Y", "[Axis] Autoscale Z"] ("Events")
            n123 = Bundle By Name(cluster=w238, "Z Scale.Z Scale.Scale Fit"=w236) -> (w237:T1)
          }
        }
        n124 = property on="Minimum" class="DigNum (strict)"("Disabled"=w220) -> ()  [unwired: 2 in, 2 out]
        n125 = property on="Maximum" class="DigNum (strict)"("Disabled"=w220) -> ()  [unwired: 2 in, 2 out]
      }
      event "Autoscale flag": Value Change {
        n126 = event-data() -> ()  [unwired: 1 in, 1 out]
        n127 = local read "Axes"() -> (w245:u16)
        n128 = case shown="0, Default" w245 {
          tunnel: w244 -> [w247 w250 w253]
          tunnel: [w248 w251 w254] -> w243
          tunnel: [w247 w250 w253] -> w242
          tunnel: [w246 w249 w252] -> w241
          frame 0, Default {
            n129 = Unbundle By Name(w247) -> ("X Scale.X Scale.Range.Minimum"=w248:dbl, "X Scale.X Scale.Range.Maximum"=w246:dbl)
          }
          frame 1 {
            n130 = Unbundle By Name(w250) -> ("Y Scale.Y Scale.Range.Minimum"=w251:dbl, "Y Scale.Y Scale.Range.Maximum"=w249:dbl)
          }
          frame 2 {
            n131 = Unbundle By Name(w253) -> ("Z Scale.Z Scale.Range.Minimum"=w254:dbl, "Z Scale.Z Scale.Range.Maximum"=w252:dbl)
          }
        }
        n132 = local write "Minimum"(w243) -> ()
        n133 = local write "Maximum"(w241) -> ()
        n134 = local write "Autoscale flag"(FALSE ("Autoscale flag")) -> ()
      }
      event "Digits", "Hide trailing zeros", "Precision Type", "Type": Value Change {
        n135 = event-data() -> ()  [unwired: 1 in, 1 out]
        n136 = local read "Apply to"() -> (w255:u16)
        n137 = call <vilib>:"svx_Colormap Digit Set.vi"("trailing zeros"="Hide trailing zeros", "Precision Type"="Precision Type", "Digits"="Digits", "Type"="Type") -> ("Fstring"=w258:string)  [unwired: 7 in]
        n138 = case shown="0, Default" w255 {
          tunnel: w260 -> [w268 w272 w276]
          tunnel: [w267 w271 w275] -> w259
          tunnel: w258 -> [w266 w270 w274]
          tunnel: [w265 w269 w273] -> w257
          frame 0, Default {
            w265 = T11[] [enum."[Axis] X FString"] items=["None", "[Axis] X Range", "[Axis] Y Range", "[Axis] Z Range", "[Axis] Range", "[Axis] X FString", "[Axis] Y FString", "[Axis] Z FString", "[Axis] X Name", "[Axis] X ScaleVis", "[Axis] X NameVis", "[Axis] Y Name", "[Axis] Y ScaleVis", "[Axis] Y NameVis", "[Axis] Z Name", "[Axis] Z ScaleVis", "[Axis] Z NameVis", "[Image] Line", "[Axis] Z Interp", "[Data] Update", "[Layout] Resize", "[ColorTable] Ignore Array", "[Legend] ScaleVis", "[Legend] GPVis", "[Legend] CPVis", "[Smooth] Update", "[Cursor] Update", "[Plot Area] Colors", "[Size] Minimum", "[Annotation] Update", "[Properties Dialog]", "[Axis] Autoscale X", "[Axis] Autoscale Y", "[Axis] Autoscale Z"] ("Events")
            n139 = Bundle By Name(cluster=w268, "X Scale.format string"=w266) -> (w267:T1)
          }
          frame 1 {
            w269 = T11[] [enum."[Axis] Y FString"] items=["None", "[Axis] X Range", "[Axis] Y Range", "[Axis] Z Range", "[Axis] Range", "[Axis] X FString", "[Axis] Y FString", "[Axis] Z FString", "[Axis] X Name", "[Axis] X ScaleVis", "[Axis] X NameVis", "[Axis] Y Name", "[Axis] Y ScaleVis", "[Axis] Y NameVis", "[Axis] Z Name", "[Axis] Z ScaleVis", "[Axis] Z NameVis", "[Image] Line", "[Axis] Z Interp", "[Data] Update", "[Layout] Resize", "[ColorTable] Ignore Array", "[Legend] ScaleVis", "[Legend] GPVis", "[Legend] CPVis", "[Smooth] Update", "[Cursor] Update", "[Plot Area] Colors", "[Size] Minimum", "[Annotation] Update", "[Properties Dialog]", "[Axis] Autoscale X", "[Axis] Autoscale Y", "[Axis] Autoscale Z"] ("Events")
            n140 = Bundle By Name(cluster=w272, "Y Scale.format string"=w270) -> (w271:T1)
          }
          frame 2 {
            w273 = T11[] [enum."[Axis] Z FString"] items=["None", "[Axis] X Range", "[Axis] Y Range", "[Axis] Z Range", "[Axis] Range", "[Axis] X FString", "[Axis] Y FString", "[Axis] Z FString", "[Axis] X Name", "[Axis] X ScaleVis", "[Axis] X NameVis", "[Axis] Y Name", "[Axis] Y ScaleVis", "[Axis] Y NameVis", "[Axis] Z Name", "[Axis] Z ScaleVis", "[Axis] Z NameVis", "[Image] Line", "[Axis] Z Interp", "[Data] Update", "[Layout] Resize", "[ColorTable] Ignore Array", "[Legend] ScaleVis", "[Legend] GPVis", "[Legend] CPVis", "[Smooth] Update", "[Cursor] Update", "[Plot Area] Colors", "[Size] Minimum", "[Annotation] Update", "[Properties Dialog]", "[Axis] Autoscale X", "[Axis] Autoscale Y", "[Axis] Autoscale Z"] ("Events")
            n141 = Bundle By Name(cluster=w276, "Z Scale.format string"=w274) -> (w275:T1)
          }
        }
      }
      event "Apply to": Value Change {
        n142 = event-data() -> ("NewVal"=w283:u16)  [unwired: 1 in]
        n143 = case shown="0, Default" w283 {
          tunnel: w284 -> [w286 w288 w290]
          tunnel: [w285 w287 w289] -> w278
          frame 0, Default {
            n144 = Unbundle By Name(w286) -> ("X Scale.format string"=w285:string)
          }
          frame 1 {
            n145 = Unbundle By Name(w288) -> ("Y Scale.format string"=w287:string)
          }
          frame 2 {
            n146 = Unbundle By Name(w290) -> ("Z Scale.format string"=w289:string)
          }
        }
        n147 = call <vilib>:"svx_Colormap Digit display.vi"("Format string"=w278) -> ("trailing zeros"=w279:bool, "Precision Type"=w280:u16, "Digits"=w281:u8, "Type"=w282:i32)  [unwired: 7 in]
        n148 = local write "Hide trailing zeros"(w279) -> ()
        n149 = local write "Precision Type"(w280) -> ()
        n150 = local write "Digits"(w281) -> ()
        n151 = local write "Type"(w282) -> ()
      }
      event "Frequencies": Shortcut Menu Activation? {
        n152 = event-data() -> ("MenuRef"=w292:refnum<k9>)  [unwired: 1 in]
        n153 = for {
          tunnel: w292 -> [w301]
          tunnel: "Menu" -> [w298] mode=indexing
          n154 = Unbundle By Name(w298) -> ("menu tag"=w297:string, "item names"=w295:string, "item tags"=w296:string)
          n155 = Insert Menu Items(5:w297, 7:w296, 8:w295, 9:w301) -> (3:w300:refnum<k9>)  [unwired: 2 in, 2 out]
          n156 = Set Menu Item Info(6:FALSE ("checked"), 7:w296, 10:w295, 11:w300) -> ()  [unwired: 3 in, 2 out]
        }
        n157 = event-data() -> ()  [unwired: 2 in, 1 out]
      }
      event "Frequencies": Shortcut Menu Selection (User) {
        w305 = T11[] [enum."[Image] Line"] items=["None", "[Axis] X Range", "[Axis] Y Range", "[Axis] Z Range", "[Axis] Range", "[Axis] X FString", "[Axis] Y FString", "[Axis] Z FString", "[Axis] X Name", "[Axis] X ScaleVis", "[Axis] X NameVis", "[Axis] Y Name", "[Axis] Y ScaleVis", "[Axis] Y NameVis", "[Axis] Z Name", "[Axis] Z ScaleVis", "[Axis] Z NameVis", "[Image] Line", "[Axis] Z Interp", "[Data] Update", "[Layout] Resize", "[ColorTable] Ignore Array", "[Legend] ScaleVis", "[Legend] GPVis", "[Legend] CPVis", "[Smooth] Update", "[Cursor] Update", "[Plot Area] Colors", "[Size] Minimum", "[Annotation] Update", "[Properties Dialog]", "[Axis] Autoscale X", "[Axis] Autoscale Y", "[Axis] Autoscale Z"] ("Events")
        n158 = event-data() -> ("ItemTag"=w307:string)  [unwired: 1 in]
        n159 = case shown="\"USER_SC_DELETE_ELEMENT\"" w307 {
          tunnel: [w308 dbl[] []] -> w304
          frame "USER_SC_DELETE_ELEMENT" {
            n160 = local read "Frequencies"() -> (w309:dbl[])
            n161 = property on="Frequencies" class="Arr (strict)"() -> ("Array Element.Value"=w313:variant, "Index Values"=w312:u32[])  [unwired: 2 in, 2 out]
            n162 = Variant To Data(type=0.0, Variant=w313) -> (data=w311:dbl)  [unwired: 1 in, 1 out]
            n163 = Index Array(array=w312) -> (element=w310:u32)  [unwired: 1 in]
            n164 = Search 1D Array(1D array=w309, element=w311, start index (0)=w310) -> (index of element=w314:i32)
            n165 = Delete From Array(array=w309, length=1, index=w314) -> (array with subset deleted=w308:dbl[])  [unwired: 1 out]
          }
          frame "USER_SC_DELETE_ALL", Default {
          }
        }
        n166 = local write "Frequencies"(w304) -> ()
        n167 = Bundle By Name(cluster=w303, "Frequency"=w304) -> (w302:T1)
      }
      event "Frequencies": Value Change {
        w318 = T11[] [enum."[Image] Line"] items=["None", "[Axis] X Range", "[Axis] Y Range", "[Axis] Z Range", "[Axis] Range", "[Axis] X FString", "[Axis] Y FString", "[Axis] Z FString", "[Axis] X Name", "[Axis] X ScaleVis", "[Axis] X NameVis", "[Axis] Y Name", "[Axis] Y ScaleVis", "[Axis] Y NameVis", "[Axis] Z Name", "[Axis] Z ScaleVis", "[Axis] Z NameVis", "[Image] Line", "[Axis] Z Interp", "[Data] Update", "[Layout] Resize", "[ColorTable] Ignore Array", "[Legend] ScaleVis", "[Legend] GPVis", "[Legend] CPVis", "[Smooth] Update", "[Cursor] Update", "[Plot Area] Colors", "[Size] Minimum", "[Annotation] Update", "[Properties Dialog]", "[Axis] Autoscale X", "[Axis] Autoscale Y", "[Axis] Autoscale Z"] ("Events")
        n168 = event-data() -> ("NewVal"=w321:dbl[])  [unwired: 1 in]
        n169 = Bundle By Name(cluster=w322, "Frequency"=w321) -> (w320:T1)
      }
      event "Orders": Shortcut Menu Activation? {
        n170 = event-data() -> ("MenuRef"=w325:refnum<k9>)  [unwired: 1 in]
        n171 = local read "Menu"() -> (w326:T3)
        n172 = for {
          tunnel: w325 -> [w333]
          tunnel: w326 -> [w330] mode=indexing
          n173 = Unbundle By Name(w330) -> ("menu tag"=w329:string, "item names"=w327:string, "item tags"=w328:string)
          n174 = Insert Menu Items(5:w329, 7:w328, 8:w327, 9:w333) -> (3:w332:refnum<k9>)  [unwired: 2 in, 2 out]
          n175 = Set Menu Item Info(6:FALSE ("checked"), 7:w328, 10:w327, 11:w332) -> ()  [unwired: 3 in, 2 out]
        }
        n176 = event-data() -> ()  [unwired: 2 in, 1 out]
      }
      event "Orders": Shortcut Menu Selection (User) {
        w338 = T11[] [enum."[Image] Line"] items=["None", "[Axis] X Range", "[Axis] Y Range", "[Axis] Z Range", "[Axis] Range", "[Axis] X FString", "[Axis] Y FString", "[Axis] Z FString", "[Axis] X Name", "[Axis] X ScaleVis", "[Axis] X NameVis", "[Axis] Y Name", "[Axis] Y ScaleVis", "[Axis] Y NameVis", "[Axis] Z Name", "[Axis] Z ScaleVis", "[Axis] Z NameVis", "[Image] Line", "[Axis] Z Interp", "[Data] Update", "[Layout] Resize", "[ColorTable] Ignore Array", "[Legend] ScaleVis", "[Legend] GPVis", "[Legend] CPVis", "[Smooth] Update", "[Cursor] Update", "[Plot Area] Colors", "[Size] Minimum", "[Annotation] Update", "[Properties Dialog]", "[Axis] Autoscale X", "[Axis] Autoscale Y", "[Axis] Autoscale Z"] ("Events")
        n177 = event-data() -> ("ItemTag"=w339:string)  [unwired: 1 in]
        n178 = case shown="\"USER_SC_DELETE_ELEMENT\"" w339 {
          tunnel: [w340 dbl[] []] -> w335
          frame "USER_SC_DELETE_ELEMENT" {
            n179 = local read "Orders"() -> (w345:dbl[])
            n180 = property on="Orders" class="Arr (strict)"() -> ("Array Element.Value"=w341:variant, "Index Values"=w342:u32[])  [unwired: 2 in, 2 out]
            n181 = Variant To Data(type=0.0, Variant=w341) -> (data=w347:dbl)  [unwired: 1 in, 1 out]
            n182 = Index Array(array=w342) -> (element=w346:u32)  [unwired: 1 in]
            n183 = Search 1D Array(1D array=w345, element=w347, start index (0)=w346) -> (index of element=w343:i32)
            n184 = Delete From Array(array=w345, length=1, index=w343) -> (array with subset deleted=w340:dbl[])  [unwired: 1 out]
          }
          frame "USER_SC_DELETE_ALL", Default {
          }
        }
        n185 = local write "Orders"(w335) -> ()
        n186 = Bundle By Name(cluster=w336, "Orders"=w335) -> (w334:T1)
      }
      event "Orders": Value Change {
        w350 = T11[] [enum."[Image] Line"] items=["None", "[Axis] X Range", "[Axis] Y Range", "[Axis] Z Range", "[Axis] Range", "[Axis] X FString", "[Axis] Y FString", "[Axis] Z FString", "[Axis] X Name", "[Axis] X ScaleVis", "[Axis] X NameVis", "[Axis] Y Name", "[Axis] Y ScaleVis", "[Axis] Y NameVis", "[Axis] Z Name", "[Axis] Z ScaleVis", "[Axis] Z NameVis", "[Image] Line", "[Axis] Z Interp", "[Data] Update", "[Layout] Resize", "[ColorTable] Ignore Array", "[Legend] ScaleVis", "[Legend] GPVis", "[Legend] CPVis", "[Smooth] Update", "[Cursor] Update", "[Plot Area] Colors", "[Size] Minimum", "[Annotation] Update", "[Properties Dialog]", "[Axis] Autoscale X", "[Axis] Autoscale Y", "[Axis] Autoscale Z"] ("Events")
        n187 = event-data() -> ("NewVal"=w353:dbl[])  [unwired: 1 in]
        n188 = Bundle By Name(cluster=w354, "Orders"=w353) -> (w352:T1)
      }
      event "DisplayLines": Value Change {
        w359 = T11[] [enum."[Image] Line"] items=["None", "[Axis] X Range", "[Axis] Y Range", "[Axis] Z Range", "[Axis] Range", "[Axis] X FString", "[Axis] Y FString", "[Axis] Z FString", "[Axis] X Name", "[Axis] X ScaleVis", "[Axis] X NameVis", "[Axis] Y Name", "[Axis] Y ScaleVis", "[Axis] Y NameVis", "[Axis] Z Name", "[Axis] Z ScaleVis", "[Axis] Z NameVis", "[Image] Line", "[Axis] Z Interp", "[Data] Update", "[Layout] Resize", "[ColorTable] Ignore Array", "[Legend] ScaleVis", "[Legend] GPVis", "[Legend] CPVis", "[Smooth] Update", "[Cursor] Update", "[Plot Area] Colors", "[Size] Minimum", "[Annotation] Update", "[Properties Dialog]", "[Axis] Autoscale X", "[Axis] Autoscale Y", "[Axis] Autoscale Z"] ("Events")
        n189 = event-data() -> ("NewVal"=w356:bool)  [unwired: 1 in]
        n190 = local read "Line Type"() -> (w355:u16)
        n191 = case shown="0, Default" w355 {
          tunnel: w358 -> [w363 w366]
          tunnel: [w362 w365] -> w357
          tunnel: w356 -> [w361 w364]
          frame 0, Default {
            n192 = Bundle By Name(cluster=w363, "Display Order Lines"=w361, "Display Order text"=w361) -> (w362:T1)
          }
          frame 1 {
            n193 = Bundle By Name(cluster=w366, "Display Frequency Lines"=w364, "Display Frequency text"=w364) -> (w365:T1)
          }
        }
        n194 = local write "Displaytext"(w356) -> ()
      }
      event "Displaytext": Value Change {
        w371 = T11[] [enum."[Image] Line"] items=["None", "[Axis] X Range", "[Axis] Y Range", "[Axis] Z Range", "[Axis] Range", "[Axis] X FString", "[Axis] Y FString", "[Axis] Z FString", "[Axis] X Name", "[Axis] X ScaleVis", "[Axis] X NameVis", "[Axis] Y Name", "[Axis] Y ScaleVis", "[Axis] Y NameVis", "[Axis] Z Name", "[Axis] Z ScaleVis", "[Axis] Z NameVis", "[Image] Line", "[Axis] Z Interp", "[Data] Update", "[Layout] Resize", "[ColorTable] Ignore Array", "[Legend] ScaleVis", "[Legend] GPVis", "[Legend] CPVis", "[Smooth] Update", "[Cursor] Update", "[Plot Area] Colors", "[Size] Minimum", "[Annotation] Update", "[Properties Dialog]", "[Axis] Autoscale X", "[Axis] Autoscale Y", "[Axis] Autoscale Z"] ("Events")
        n195 = event-data() -> ("NewVal"=w368:bool)  [unwired: 1 in]
        n196 = local read "Line Type"() -> (w367:u16)
        n197 = case shown="0, Default" w367 {
          tunnel: w370 -> [w375 w378]
          tunnel: [w374 w377] -> w369
          tunnel: w368 -> [w373 w376]
          frame 0, Default {
            n198 = Bundle By Name(cluster=w375, "Display Order text"=w373) -> (w374:T1)
          }
          frame 1 {
            n199 = Bundle By Name(cluster=w378, "Display Frequency text"=w376) -> (w377:T1)
          }
        }
      }
      event "Show scale": Value Change {
        n200 = event-data() -> ("NewVal"=w383:bool)  [unwired: 1 in]
        n201 = local read "Axes"() -> (w384:u16)
        n202 = case shown="0, Default" w384 {
          tunnel: w383 -> [w386 w390 w394]
          tunnel: w381 -> [w388 w392 w396]
          tunnel: [w387 w391 w395] -> w380
          tunnel: [w385 w389 w393] -> w379
          frame 0, Default {
            w385 = T11[] [enum."[Axis] X ScaleVis"] items=["None", "[Axis] X Range", "[Axis] Y Range", "[Axis] Z Range", "[Axis] Range", "[Axis] X FString", "[Axis] Y FString", "[Axis] Z FString", "[Axis] X Name", "[Axis] X ScaleVis", "[Axis] X NameVis", "[Axis] Y Name", "[Axis] Y ScaleVis", "[Axis] Y NameVis", "[Axis] Z Name", "[Axis] Z ScaleVis", "[Axis] Z NameVis", "[Image] Line", "[Axis] Z Interp", "[Data] Update", "[Layout] Resize", "[ColorTable] Ignore Array", "[Legend] ScaleVis", "[Legend] GPVis", "[Legend] CPVis", "[Smooth] Update", "[Cursor] Update", "[Plot Area] Colors", "[Size] Minimum", "[Annotation] Update", "[Properties Dialog]", "[Axis] Autoscale X", "[Axis] Autoscale Y", "[Axis] Autoscale Z"] ("Events")
            n203 = Bundle By Name(cluster=w388, "X Scale.Visible"=w386) -> (w387:T1)
          }
          frame 1 {
            w389 = T11[] [enum."[Axis] Y ScaleVis"] items=["None", "[Axis] X Range", "[Axis] Y Range", "[Axis] Z Range", "[Axis] Range", "[Axis] X FString", "[Axis] Y FString", "[Axis] Z FString", "[Axis] X Name", "[Axis] X ScaleVis", "[Axis] X NameVis", "[Axis] Y Name", "[Axis] Y ScaleVis", "[Axis] Y NameVis", "[Axis] Z Name", "[Axis] Z ScaleVis", "[Axis] Z NameVis", "[Image] Line", "[Axis] Z Interp", "[Data] Update", "[Layout] Resize", "[ColorTable] Ignore Array", "[Legend] ScaleVis", "[Legend] GPVis", "[Legend] CPVis", "[Smooth] Update", "[Cursor] Update", "[Plot Area] Colors", "[Size] Minimum", "[Annotation] Update", "[Properties Dialog]", "[Axis] Autoscale X", "[Axis] Autoscale Y", "[Axis] Autoscale Z"] ("Events")
            n204 = Bundle By Name(cluster=w392, "Y Scale.Visible"=w390) -> (w391:T1)
          }
          frame 2 {
            w393 = T11[] [enum."[Axis] Z ScaleVis"] items=["None", "[Axis] X Range", "[Axis] Y Range", "[Axis] Z Range", "[Axis] Range", "[Axis] X FString", "[Axis] Y FString", "[Axis] Z FString", "[Axis] X Name", "[Axis] X ScaleVis", "[Axis] X NameVis", "[Axis] Y Name", "[Axis] Y ScaleVis", "[Axis] Y NameVis", "[Axis] Z Name", "[Axis] Z ScaleVis", "[Axis] Z NameVis", "[Image] Line", "[Axis] Z Interp", "[Data] Update", "[Layout] Resize", "[ColorTable] Ignore Array", "[Legend] ScaleVis", "[Legend] GPVis", "[Legend] CPVis", "[Smooth] Update", "[Cursor] Update", "[Plot Area] Colors", "[Size] Minimum", "[Annotation] Update", "[Properties Dialog]", "[Axis] Autoscale X", "[Axis] Autoscale Y", "[Axis] Autoscale Z"] ("Events")
            n205 = Bundle By Name(cluster=w396, "Z Scale.Visible"=w394) -> (w395:T1)
          }
        }
      }
      event "Show scale label": Value Change {
        n206 = event-data() -> ("NewVal"=w400:bool)  [unwired: 1 in]
        n207 = local read "Axes"() -> (w397:u16)
        n208 = case shown="0, Default" w397 {
          tunnel: w400 -> [w404 w408 w412]
          tunnel: w402 -> [w406 w410 w414]
          tunnel: [w405 w409 w413] -> w401
          tunnel: [w403 w407 w411] -> w399
          frame 0, Default {
            w403 = T11[] [enum."[Axis] X NameVis"] items=["None", "[Axis] X Range", "[Axis] Y Range", "[Axis] Z Range", "[Axis] Range", "[Axis] X FString", "[Axis] Y FString", "[Axis] Z FString", "[Axis] X Name", "[Axis] X ScaleVis", "[Axis] X NameVis", "[Axis] Y Name", "[Axis] Y ScaleVis", "[Axis] Y NameVis", "[Axis] Z Name", "[Axis] Z ScaleVis", "[Axis] Z NameVis", "[Image] Line", "[Axis] Z Interp", "[Data] Update", "[Layout] Resize", "[ColorTable] Ignore Array", "[Legend] ScaleVis", "[Legend] GPVis", "[Legend] CPVis", "[Smooth] Update", "[Cursor] Update", "[Plot Area] Colors", "[Size] Minimum", "[Annotation] Update", "[Properties Dialog]", "[Axis] Autoscale X", "[Axis] Autoscale Y", "[Axis] Autoscale Z"] ("Events")
            n209 = Bundle By Name(cluster=w406, "X Scale.Label Visible"=w404) -> (w405:T1)
          }
          frame 1 {
            w407 = T11[] [enum."[Axis] Y NameVis"] items=["None", "[Axis] X Range", "[Axis] Y Range", "[Axis] Z Range", "[Axis] Range", "[Axis] X FString", "[Axis] Y FString", "[Axis] Z FString", "[Axis] X Name", "[Axis] X ScaleVis", "[Axis] X NameVis", "[Axis] Y Name", "[Axis] Y ScaleVis", "[Axis] Y NameVis", "[Axis] Z Name", "[Axis] Z ScaleVis", "[Axis] Z NameVis", "[Image] Line", "[Axis] Z Interp", "[Data] Update", "[Layout] Resize", "[ColorTable] Ignore Array", "[Legend] ScaleVis", "[Legend] GPVis", "[Legend] CPVis", "[Smooth] Update", "[Cursor] Update", "[Plot Area] Colors", "[Size] Minimum", "[Annotation] Update", "[Properties Dialog]", "[Axis] Autoscale X", "[Axis] Autoscale Y", "[Axis] Autoscale Z"] ("Events")
            n210 = Bundle By Name(cluster=w410, "Y Scale.Label Visible"=w408) -> (w409:T1)
          }
          frame 2 {
            w411 = T11[] [enum."[Axis] Z NameVis"] items=["None", "[Axis] X Range", "[Axis] Y Range", "[Axis] Z Range", "[Axis] Range", "[Axis] X FString", "[Axis] Y FString", "[Axis] Z FString", "[Axis] X Name", "[Axis] X ScaleVis", "[Axis] X NameVis", "[Axis] Y Name", "[Axis] Y ScaleVis", "[Axis] Y NameVis", "[Axis] Z Name", "[Axis] Z ScaleVis", "[Axis] Z NameVis", "[Image] Line", "[Axis] Z Interp", "[Data] Update", "[Layout] Resize", "[ColorTable] Ignore Array", "[Legend] ScaleVis", "[Legend] GPVis", "[Legend] CPVis", "[Smooth] Update", "[Cursor] Update", "[Plot Area] Colors", "[Size] Minimum", "[Annotation] Update", "[Properties Dialog]", "[Axis] Autoscale X", "[Axis] Autoscale Y", "[Axis] Autoscale Z"] ("Events")
            n211 = Bundle By Name(cluster=w414, "Z Scale.Label Visible"=w412) -> (w413:T1)
          }
        }
      }
      event "Minimum", "Maximum": Value Change {
        n212 = local read "Axes"() -> (w419:u16)
        n213 = event-data() -> ()  [unwired: 1 in, 1 out]
        n214 = Max & Min(x="Minimum", y="Maximum") -> (max(x,y)=w416:dbl, min(x,y)=w415:dbl)
        n215 = case shown="1" w419 {
          tunnel: w423 -> [w428 w433 w438]
          tunnel: [w427 w432 w437] -> w422
          tunnel: [w426 w431 w436] -> w421
          tunnel: w416 -> [w425 w430 w435]
          tunnel: w415 -> [w424 w429 w434]
          frame 0, Default {
            w426 = T11[] [enum."[Axis] X Range"] items=["None", "[Axis] X Range", "[Axis] Y Range", "[Axis] Z Range", "[Axis] Range", "[Axis] X FString", "[Axis] Y FString", "[Axis] Z FString", "[Axis] X Name", "[Axis] X ScaleVis", "[Axis] X NameVis", "[Axis] Y Name", "[Axis] Y ScaleVis", "[Axis] Y NameVis", "[Axis] Z Name", "[Axis] Z ScaleVis", "[Axis] Z NameVis", "[Image] Line", "[Axis] Z Interp", "[Data] Update", "[Layout] Resize", "[ColorTable] Ignore Array", "[Legend] ScaleVis", "[Legend] GPVis", "[Legend] CPVis", "[Smooth] Update", "[Cursor] Update", "[Plot Area] Colors", "[Size] Minimum", "[Annotation] Update", "[Properties Dialog]", "[Axis] Autoscale X", "[Axis] Autoscale Y", "[Axis] Autoscale Z"] ("Events")
            n216 = Bundle By Name(cluster=w428, "X Scale.X Scale.Range.Maximum"=w425, "X Scale.X Scale.Range.Minimum"=w424) -> (w427:T1)
          }
          frame 1 {
            w431 = T11[] [enum."[Axis] Y Range"] items=["None", "[Axis] X Range", "[Axis] Y Range", "[Axis] Z Range", "[Axis] Range", "[Axis] X FString", "[Axis] Y FString", "[Axis] Z FString", "[Axis] X Name", "[Axis] X ScaleVis", "[Axis] X NameVis", "[Axis] Y Name", "[Axis] Y ScaleVis", "[Axis] Y NameVis", "[Axis] Z Name", "[Axis] Z ScaleVis", "[Axis] Z NameVis", "[Image] Line", "[Axis] Z Interp", "[Data] Update", "[Layout] Resize", "[ColorTable] Ignore Array", "[Legend] ScaleVis", "[Legend] GPVis", "[Legend] CPVis", "[Smooth] Update", "[Cursor] Update", "[Plot Area] Colors", "[Size] Minimum", "[Annotation] Update", "[Properties Dialog]", "[Axis] Autoscale X", "[Axis] Autoscale Y", "[Axis] Autoscale Z"] ("Events")
            n217 = Bundle By Name(cluster=w433, "Y Scale.Y Scale.Range.Maximum"=w430, "Y Scale.Y Scale.Range.Minimum"=w429) -> (w432:T1)
          }
          frame 2 {
            w436 = T11[] [enum."[Axis] Z Range"] items=["None", "[Axis] X Range", "[Axis] Y Range", "[Axis] Z Range", "[Axis] Range", "[Axis] X FString", "[Axis] Y FString", "[Axis] Z FString", "[Axis] X Name", "[Axis] X ScaleVis", "[Axis] X NameVis", "[Axis] Y Name", "[Axis] Y ScaleVis", "[Axis] Y NameVis", "[Axis] Z Name", "[Axis] Z ScaleVis", "[Axis] Z NameVis", "[Image] Line", "[Axis] Z Interp", "[Data] Update", "[Layout] Resize", "[ColorTable] Ignore Array", "[Legend] ScaleVis", "[Legend] GPVis", "[Legend] CPVis", "[Smooth] Update", "[Cursor] Update", "[Plot Area] Colors", "[Size] Minimum", "[Annotation] Update", "[Properties Dialog]", "[Axis] Autoscale X", "[Axis] Autoscale Y", "[Axis] Autoscale Z"] ("Events")
            n218 = Bundle By Name(cluster=w438, "Z Scale.Z Scale.Range.Maximum"=w435, "Z Scale.Z Scale.Range.Minimum"=w434) -> (w437:T1)
          }
        }
        n219 = local write "Minimum"(w415) -> ()
        n220 = local write "Maximum"(w416) -> ()
      }
      event "Interpolate color": Value Change {
        w439 = T11[] [enum."[Axis] Z Interp"] items=["None", "[Axis] X Range", "[Axis] Y Range", "[Axis] Z Range", "[Axis] Range", "[Axis] X FString", "[Axis] Y FString", "[Axis] Z FString", "[Axis] X Name", "[Axis] X ScaleVis", "[Axis] X NameVis", "[Axis] Y Name", "[Axis] Y ScaleVis", "[Axis] Y NameVis", "[Axis] Z Name", "[Axis] Z ScaleVis", "[Axis] Z NameVis", "[Image] Line", "[Axis] Z Interp", "[Data] Update", "[Layout] Resize", "[ColorTable] Ignore Array", "[Legend] ScaleVis", "[Legend] GPVis", "[Legend] CPVis", "[Smooth] Update", "[Cursor] Update", "[Plot Area] Colors", "[Size] Minimum", "[Annotation] Update", "[Properties Dialog]", "[Axis] Autoscale X", "[Axis] Autoscale Y", "[Axis] Autoscale Z"] ("Events")
        n221 = event-data() -> ("NewVal"=w441:bool)  [unwired: 1 in]
        n222 = Bundle By Name(cluster=w443, "Z Scale.Z Scale.Interpolate Color"=w441) -> (w442:T1)
      }
      event "Label": Value Change {
        n223 = event-data() -> ("NewVal"=w444:bool)  [unwired: 1 in]
        n224 = Select(t=u8 0 ("Disabled"), s=w444, f=u8 2) -> (s? t:f=w449:u8)
        n225 = property class="Ctl"(reference=w448, "Label.Visible"=w444) -> ()  [unwired: 1 in, 2 out]
        n226 = Bundle By Name(cluster=w446, "Label.Visible"=w444) -> (w445:T8)
        n227 = property on="Label Text" class="Str"("Disabled"=w449) -> ()  [unwired: 2 in, 2 out]
      }
      event "Label Text": Value Change {
        n228 = event-data() -> ("NewVal"=w452:string)  [unwired: 1 in]
        n229 = Bundle By Name(cluster=w454, "Label.Text"=w452) -> (w453:T8)
        n230 = property class="Ctl"(reference=w456, "Label.Text"=w452) -> ()  [unwired: 1 in, 2 out]
      }
      event "Caption": Value Change {
        n231 = event-data() -> ("NewVal"=w457:bool)  [unwired: 1 in]
        n232 = Select(t=u8 0 ("Disabled"), s=w457, f=u8 2) -> (s? t:f=w462:u8)
        n233 = property class="Ctl"(reference=w461, "Caption.Visible"=w457) -> ()  [unwired: 1 in, 2 out]
        n234 = Bundle By Name(cluster=w459, "Caption.Visible"=w457) -> (w458:T8)
        n235 = property on="Caption" class="Str"("Disabled"=w462) -> ()  [unwired: 2 in, 2 out]
      }
      event "Caption": Value Change {
        n236 = event-data() -> ("NewVal"=w465:string)  [unwired: 1 in]
        n237 = Bundle By Name(cluster=w467, "Caption.Text"=w465) -> (w466:T8)
        n238 = property class="Ctl"(reference=w469, "Caption.Text"=w465) -> ()  [unwired: 1 in, 2 out]
      }
      event "Enable State": Value Change {
        n239 = event-data() -> ("NewVal"=w471:T6)  [unwired: 1 in]
        n240 = To Unsigned Byte Integer(number=w471) -> (unsigned 8bit integer=w475:u8)
        n241 = Bundle By Name(cluster=w472, "Disabled"=w471) -> (w470:T8)
        n242 = property class="Ctl"(reference=w474, "Disabled"=w475) -> ()  [unwired: 1 in, 2 out]
      }
      event "Description": Value Change {
        n243 = event-data() -> ("NewVal"=w476:string)  [unwired: 1 in]
        n244 = Bundle By Name(cluster=w478, "Desc"=w476) -> (w477:T8)
        n245 = property class="Ctl"(reference=w480, "Desc"=w476) -> ()  [unwired: 1 in, 2 out]
      }
      event "Tip strip": Value Change {
        n246 = event-data() -> ("NewVal"=w481:string)  [unwired: 1 in]
        n247 = Bundle By Name(cluster=w483, "TipStrip"=w481) -> (w482:T8)
        n248 = property class="Ctl"(reference=w485, "TipStrip"=w481) -> ()  [unwired: 1 in, 2 out]
      }
      event "Style", "Line color", "Line width", "Size", "Text color", "BG color": Value Change {
        w494 = T11[] [enum."[Image] Line"] items=["None", "[Axis] X Range", "[Axis] Y Range", "[Axis] Z Range", "[Axis] Range", "[Axis] X FString", "[Axis] Y FString", "[Axis] Z FString", "[Axis] X Name", "[Axis] X ScaleVis", "[Axis] X NameVis", "[Axis] Y Name", "[Axis] Y ScaleVis", "[Axis] Y NameVis", "[Axis] Z Name", "[Axis] Z ScaleVis", "[Axis] Z NameVis", "[Image] Line", "[Axis] Z Interp", "[Data] Update", "[Layout] Resize", "[ColorTable] Ignore Array", "[Legend] ScaleVis", "[Legend] GPVis", "[Legend] CPVis", "[Smooth] Update", "[Cursor] Update", "[Plot Area] Colors", "[Size] Minimum", "[Annotation] Update", "[Properties Dialog]", "[Axis] Autoscale X", "[Axis] Autoscale Y", "[Axis] Autoscale Z"] ("Events")
        n249 = event-data() -> ()  [unwired: 1 in, 6 out]
        n250 = local read "Line Type"() -> (w493:u16)
        n251 = case shown="0" w493 {
          tunnel: w496 -> [w504 w512]
          tunnel: [w503 w511] -> w495
          tunnel: "Line width" -> [w502 w510]
          tunnel: "Style" -> [w501 w509]
          tunnel: "Line color" -> [w500 w508]
          tunnel: "Size" -> [w499 w507]
          tunnel: "Text color" -> [w498 w506]
          tunnel: "BG color" -> [w497 w505]
          frame 1, Default {
            n252 = Bundle By Name(cluster=w504, "Frequency Lineproperty.Line.Width"=w502, "Frequency Lineproperty.Line.Style"=w501, "Frequency Lineproperty.color"=w500, "Frequency Textproperty.Test size"=w499, "Frequency Textproperty.color"=w498, "Frequency Textproperty.background"=w497) -> (w503:T1)
          }
          frame 0 {
            n253 = Bundle By Name(cluster=w512, "Order Lineproperty.Line.Width"=w510, "Order Lineproperty.Line.Style"=w509, "Order Lineproperty.color"=w508, "Order Textproperty.Test size"=w507, "Order Textproperty.color"=w506, "Order Textproperty.background"=w505) -> (w511:T1)
          }
        }
      }
    }
    n254 = call <vilib>:"svx_Colormap Exec Commands.vi"("Container ref"=w80, "Colormap ref"=w84, "Events"=w82, "State in"=w86, "Data in"=w83) -> ("State out"=w85:T1)  [unwired: 6 in]
  }
  "Action" <- w16
  "State out" <- w2
